vi "xijk_automatic_read_and_guess.vi"(8 "error in":errorcluster, 11 "path in":path) -> (0 "error out":errorcluster, 3 "table out":path[](array[path]))   [LabVIEW 2010, in "xijk_automatic_read_and_guess.lvlib"]
uses:
  xijk_automatic_read_and_guess.lvlib
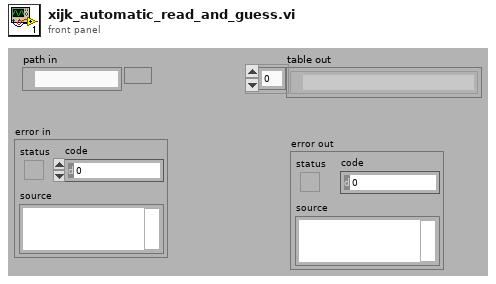
[diagram p1: front panel]
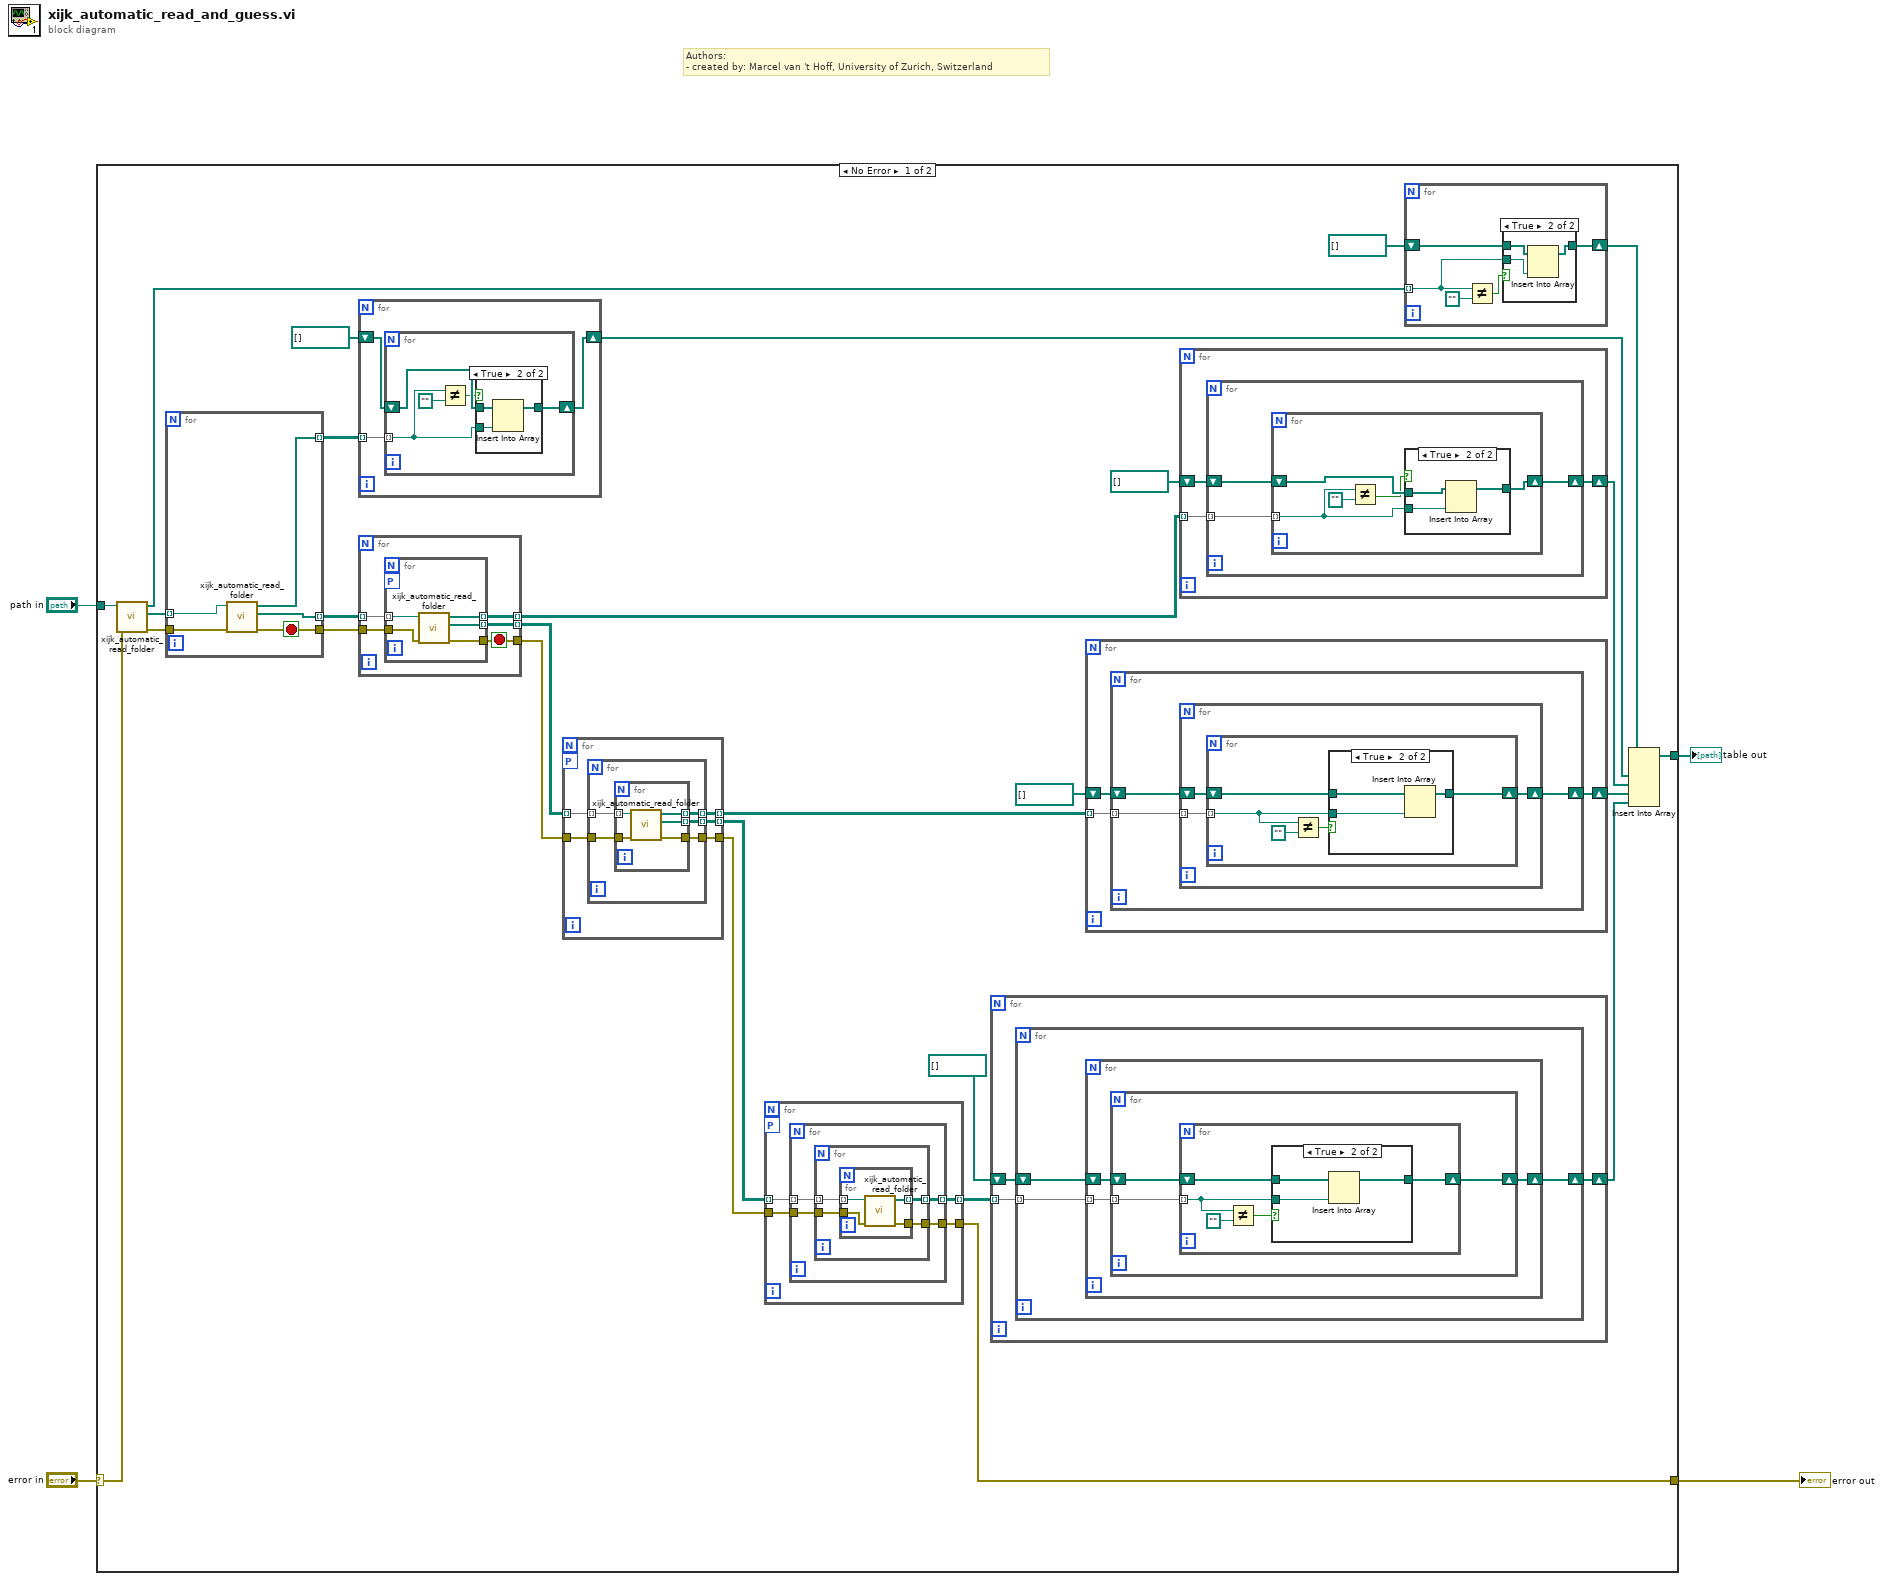
[diagram p0: block diagram]
diagram:
  # "Authors: \n- created by: Marcel van 't Hoff, University of Zurich, Switzerland"
  n1 = case shown="No Error" "error in" {
    selector: "error in" -> [w10 w153]
    tunnel: "path in" -> [w30 _]
    tunnel: [w15 _] -> w3
    tunnel: [w5 w153] -> w1
    frame No Error {
      n2 = call "xijk_automatic_read_folder.vi"("error in"=w10, "path in"=w30) -> ("error out"=w9:errorcluster, "Filenames folders"=w27:path[], "Output filenames"=w14:path[])  [unwired: 7 out]
      n3 = for {
        tunnel: w27 -> [w151] mode=indexing
        tunnel: [w152] -> w31 mode=indexing
        tunnel: [w150] -> w26 mode=indexing
        tunnel: w9 -> [w149]
        tunnel: [w148] -> w8
        stop <- w148 stop-if-true
        n4 = call "xijk_automatic_read_folder.vi"("error in"=w149, "path in"=w151) -> ("error out"=w148:errorcluster, "Filenames folders"=w152:path[], "Output filenames"=w150:path[])  [unwired: 7 out]
      }
      n5 = for {
        tunnel: w26 -> [w97] mode=indexing
        shift-right: [w95] -> w12
        shift-left: path[] [] -> [w96]
        n6 = for {
          tunnel: w97 -> [w99] mode=indexing
          shift-right: [w101] -> w95
          shift-left: w96 -> [w102]
          n7 = Not Equal?(x=w99, y=path "") -> (x != y?=w98:bool)
          n8 = case shown="True" w98 {
            tunnel: w99 -> [_ w106]
            tunnel: w102 -> [w103 w105]
            tunnel: [w103 w104] -> w101
            frame False {
            }
            frame True {
              n9 = Insert Into Array(array=w105, new element=w106) -> (w104:path[])  [unwired: 1 in]
            }
          }
        }
      }
      n10 = for {
        tunnel: w31 -> [w142] mode=indexing
        tunnel: [w141] -> w29 mode=indexing
        tunnel: [w140] -> w24 mode=indexing
        tunnel: w8 -> [w139]
        tunnel: [w138] -> w7
        stop <- w138 stop-if-true
        n11 = for {
          tunnel: w142 -> [w147] mode=indexing
          tunnel: [w146] -> w141 mode=indexing
          tunnel: [w145] -> w140 mode=indexing
          tunnel: w139 -> [w144]
          tunnel: [w143] -> w138
          workers-P: _ -> [_]
          n12 = call "xijk_automatic_read_folder.vi"("error in"=w144, "path in"=w147) -> ("error out"=w143:errorcluster, "Filenames folders"=w146:path[], "Output filenames"=w145:path[])  [unwired: 7 out]
        }
      }
      n13 = for {
        tunnel: w29 -> [w127] mode=indexing
        tunnel: [w126] -> w28 mode=indexing
        tunnel: [w125] -> w21 mode=indexing
        tunnel: w7 -> [w124]
        tunnel: [w123] -> w6
        workers-P: _ -> [_]
        n14 = for {
          tunnel: w127 -> [w132] mode=indexing
          tunnel: [w131] -> w126 mode=indexing
          tunnel: [w130] -> w125 mode=indexing
          tunnel: w124 -> [w129]
          tunnel: [w128] -> w123
          n15 = for {
            tunnel: w132 -> [w137] mode=indexing
            tunnel: [w136] -> w131 mode=indexing
            tunnel: [w135] -> w130 mode=indexing
            tunnel: w129 -> [w134]
            tunnel: [w133] -> w128
            n16 = call "xijk_automatic_read_folder.vi"("error in"=w134, "path in"=w137) -> ("error out"=w133:errorcluster, "Filenames folders"=w136:path[], "Output filenames"=w135:path[])  [unwired: 7 out]
          }
        }
      }
      n17 = for {
        tunnel: w28 -> [w110] mode=indexing
        tunnel: [w109] -> w19 mode=indexing
        tunnel: w6 -> [w108]
        tunnel: [w107] -> w5
        workers-P: _ -> [_]
        n18 = for {
          tunnel: w110 -> [w114] mode=indexing
          tunnel: [w113] -> w109 mode=indexing
          tunnel: w108 -> [w112]
          tunnel: [w111] -> w107
          n19 = for {
            tunnel: w114 -> [w118] mode=indexing
            tunnel: [w117] -> w113 mode=indexing
            tunnel: w112 -> [w116]
            tunnel: [w115] -> w111
            n20 = for {
              tunnel: w118 -> [w122] mode=indexing
              tunnel: [w121] -> w117 mode=indexing
              tunnel: w116 -> [w120]
              tunnel: [w119] -> w115
              n21 = call "xijk_automatic_read_folder.vi"("error in"=w120, "path in"=w122) -> ("error out"=w119:errorcluster, "Output filenames"=w121:path[])  [unwired: 8 out]
            }
          }
        }
      }
      n22 = for {
        shift-right: [w42] -> w16
        shift-left: path[] [] -> [w43]
        tunnel: w19 -> [w41] mode=indexing
        n23 = for {
          tunnel: w41 -> [w44] mode=indexing
          shift-right: [w46] -> w42
          shift-left: w43 -> [w45]
          n24 = for {
            tunnel: w44 -> [w49] mode=indexing
            shift-right: [w47] -> w46
            shift-left: w45 -> [w48]
            n25 = for {
              tunnel: w49 -> [w52] mode=indexing
              shift-right: [w50] -> w47
              shift-left: w48 -> [w51]
              n26 = for {
                tunnel: w52 -> [w54] mode=indexing
                shift-right: [w56] -> w50
                shift-left: w51 -> [w57]
                n27 = Not Equal?(x=w54, y=path "") -> (x != y?=w53:bool)
                n28 = case shown="True" w53 {
                  tunnel: w54 -> [_ w61]
                  tunnel: w57 -> [w58 w60]
                  tunnel: [w58 w59] -> w56
                  frame False {
                  }
                  frame True {
                    n29 = Insert Into Array(array=w60, new element=w61) -> (w59:path[])  [unwired: 1 in]
                  }
                }
              }
            }
          }
        }
      }
      n30 = for {
        tunnel: w21 -> [w62] mode=indexing
        shift-right: [w64] -> w17
        shift-left: path[] [] -> [w63]
        n31 = for {
          tunnel: w62 -> [w67] mode=indexing
          shift-right: [w65] -> w64
          shift-left: w63 -> [w66]
          n32 = for {
            tunnel: w67 -> [w70] mode=indexing
            shift-right: [w68] -> w65
            shift-left: w66 -> [w69]
            n33 = for {
              tunnel: w70 -> [w72] mode=indexing
              shift-right: [w74] -> w68
              shift-left: w69 -> [w75]
              n34 = Not Equal?(x=w72, y=path "") -> (x != y?=w71:bool)
              n35 = case shown="True" w71 {
                tunnel: w72 -> [_ w79]
                tunnel: w75 -> [w76 w78]
                tunnel: [w76 w77] -> w74
                frame False {
                }
                frame True {
                  n36 = Insert Into Array(array=w78, new element=w79) -> (w77:path[])  [unwired: 1 in]
                }
              }
            }
          }
        }
      }
      n37 = for {
        tunnel: w24 -> [w82] mode=indexing
        shift-right: [w80] -> w18
        shift-left: path[] [] -> [w81]
        n38 = for {
          tunnel: w82 -> [w85] mode=indexing
          shift-right: [w83] -> w80
          shift-left: w81 -> [w84]
          n39 = for {
            tunnel: w85 -> [w87] mode=indexing
            shift-right: [w89] -> w83
            shift-left: w84 -> [w90]
            n40 = Not Equal?(x=w87, y=path "") -> (x != y?=w86:bool)
            n41 = case shown="True" w86 {
              tunnel: w87 -> [_ w94]
              tunnel: w90 -> [w91 w93]
              tunnel: [w91 w92] -> w89
              frame False {
              }
              frame True {
                n42 = Insert Into Array(array=w93, new element=w94) -> (w92:path[])  [unwired: 1 in]
              }
            }
          }
        }
      }
      n43 = for {
        tunnel: w14 -> [w33] mode=indexing
        shift-right: [w35] -> w11
        shift-left: path[] [] -> [w36]
        n44 = Not Equal?(x=w33, y=path "") -> (x != y?=w32:bool)
        n45 = case shown="True" w32 {
          tunnel: w33 -> [_ w40]
          tunnel: w36 -> [w37 w39]
          tunnel: [w37 w38] -> w35
          frame False {
          }
          frame True {
            n46 = Insert Into Array(array=w39, new element=w40) -> (w38:path[])  [unwired: 1 in]
          }
        }
      }
      n47 = Insert Into Array(array=w11, new element #1=w12, new element #2=w18, new element #3=w17, new element #4=w16) -> (w15:path[])  [unwired: 1 in]
    }
    frame Error {
    }
  }
  "table out" <- w3
  "error out" <- w1
